vi "PID_auto.vi"() -> ()   [LabVIEW 2025]
uses:
  <vilib>/DAQmx/write.llb/DAQmx Write (Analog 1D DBL NChan 1Samp).vi
  <vilib>/DAQmx/read.llb/DAQmx Read (Analog 1D Wfm NChan NSamp).vi
  <vilib>/Analysis/baseanly.llb/Mean (DBL).vi
  <vilib>/DAQmx/create/channels.llb/DAQmx Create Channel (AO-Voltage-Basic).vi
  <vilib>/DAQmx/configure/timing.llb/DAQmx Timing (Sample Clock).vi
  <vilib>/addons/control/pid/pid.llb/PID (DBL).vi
  <vilib>/addons/control/pid/pid.llb/PID Output Rate Limiter (DBL).vi
  <vilib>/DAQmx/miscellaneous.llb/DAQmx Fill In Error Info.vi
  <resource>/objmgr/daqmx.rc
  <vilib>/addons/control/pid/NI_PID_pid.lvlib
  <vilib>/Analysis/NI_AALBase.lvlib
panel:
  out "Waveform Graph":dbl[](graph)
  out "Mass Flow Rate":dbl
  in  "SO-2":bool
  out "Upstream Temperature":dbl
  out "Inlet Temperature":dbl
  out "PID Gains Indicator":T1={"proportional gain (Kc)"=0.16, "integral time (Ti, min)"=0.0, "derivative time (Td, min)"=0.0}
  in  "Send to Target Position":dbl format="%_3g"
  in  "Emergency Valve Control":dbl format="%_3g"
  in  "Control Options":bool[](array[boolean])
  in  "Control Loop STOP":bool
  in  "Ignition":bool
  in  "SO-1":bool
  out "Valve Output Voltage":dbl format="%_3g"
  out "Time (s)":dbl
  out "error out":errorcluster
  in  "Setpoint":dbl
  out "Thrust Sensor":dbl
  out "Valve Position (%)":dbl format="%_3g"
  out "Differential Pressure":dbl
  out "Chamber Pressure":dbl
  out "Inlet Pressure":dbl
  out "Upstream Pressure":dbl
  out "Supply Pressure":dbl
  in  "Filename":path=path "C:/1. Rocket Research Project/CollectedData/Plots/TestingData.lvm"
  in  "Data Collection Enabled":bool=TRUE caption="Enable"
  in  "Data Collection STOP":bool
  in  "rate":dbl=1000.0 format="%0.2f"
  # "DATA COLLECTION"
  # "CONTROL OPERATIONS"
  # "INSTRUMENTATION"
  # "Pressure"
  # "%"
  # "Emergency Control"
  # "V"
  # "V"
  # "Manual Control"
  # "%"
  # "Auto"
  # "Temperature"
  # "Thrust"
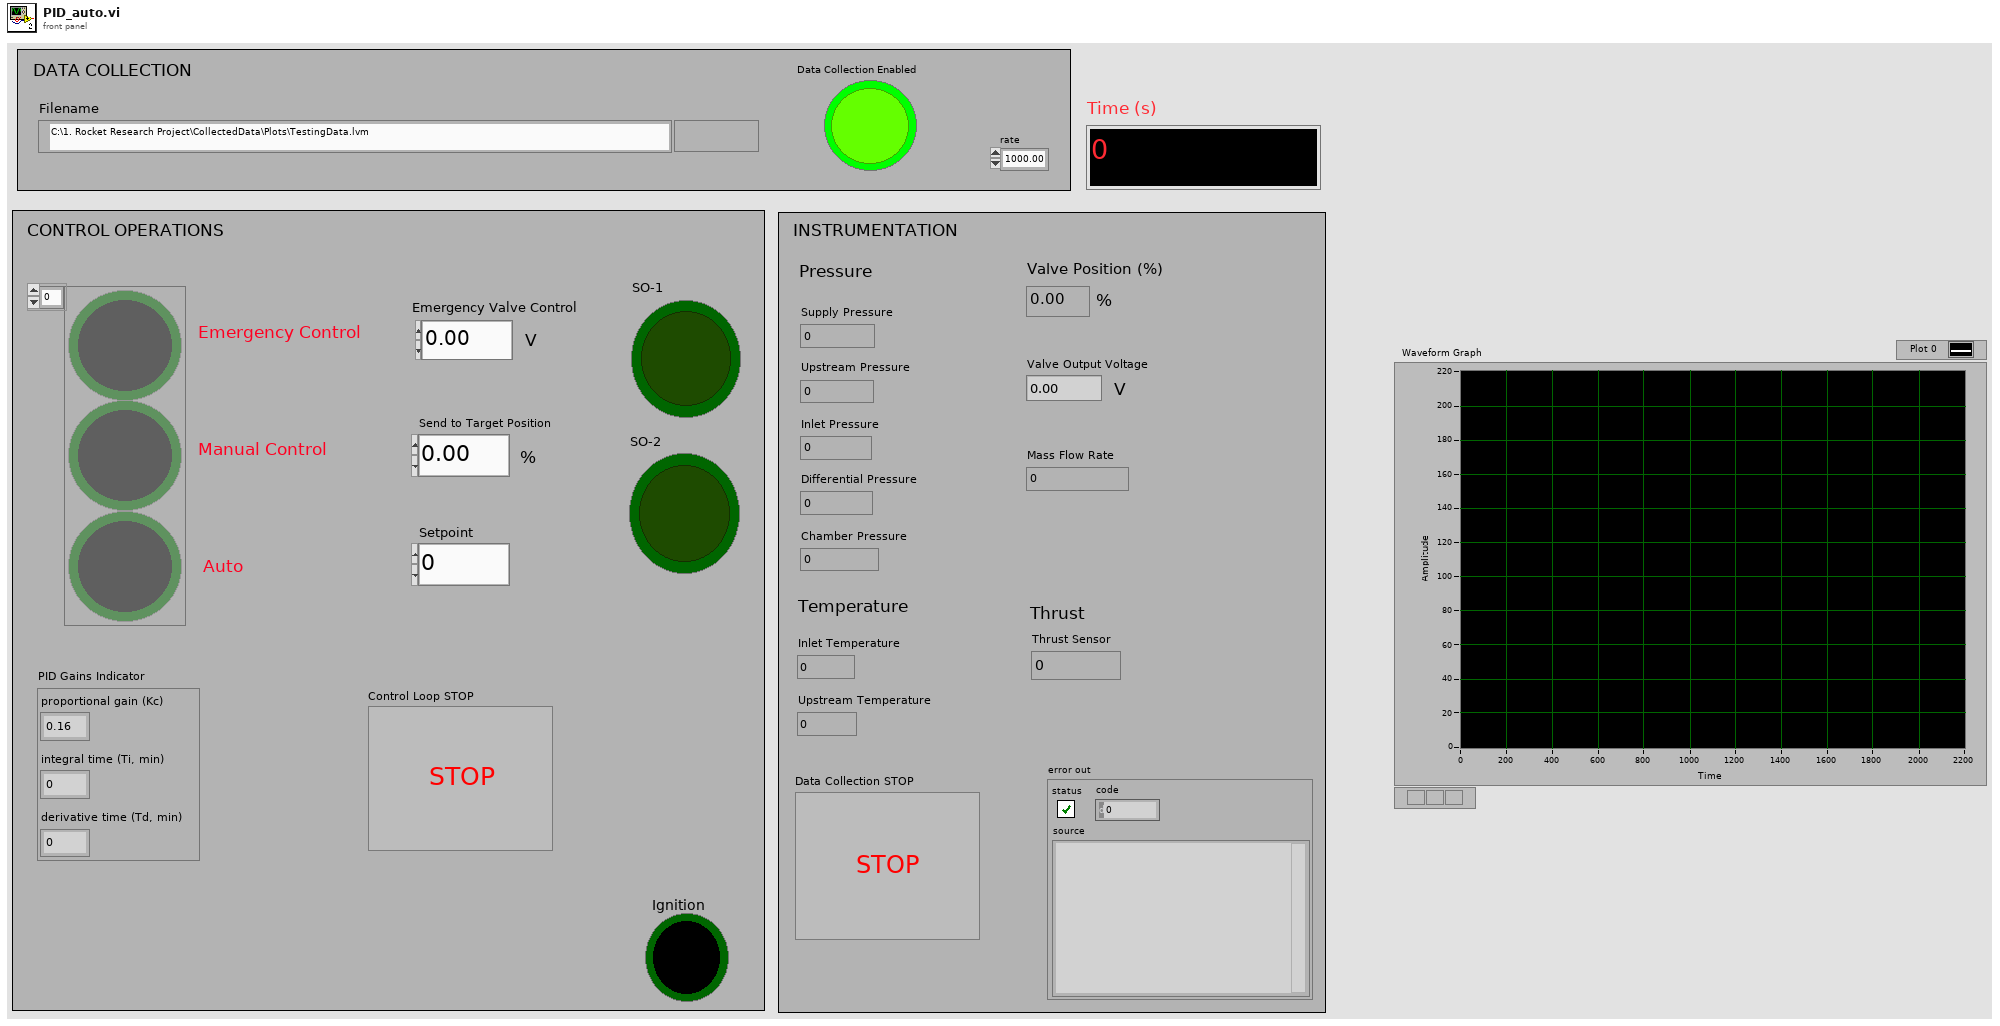
[diagram p1: front panel]
types:
  T1 = cluster{"proportional gain (Kc)":dbl, "integral time (Ti, min)":dbl, "derivative time (Td, min)":dbl}
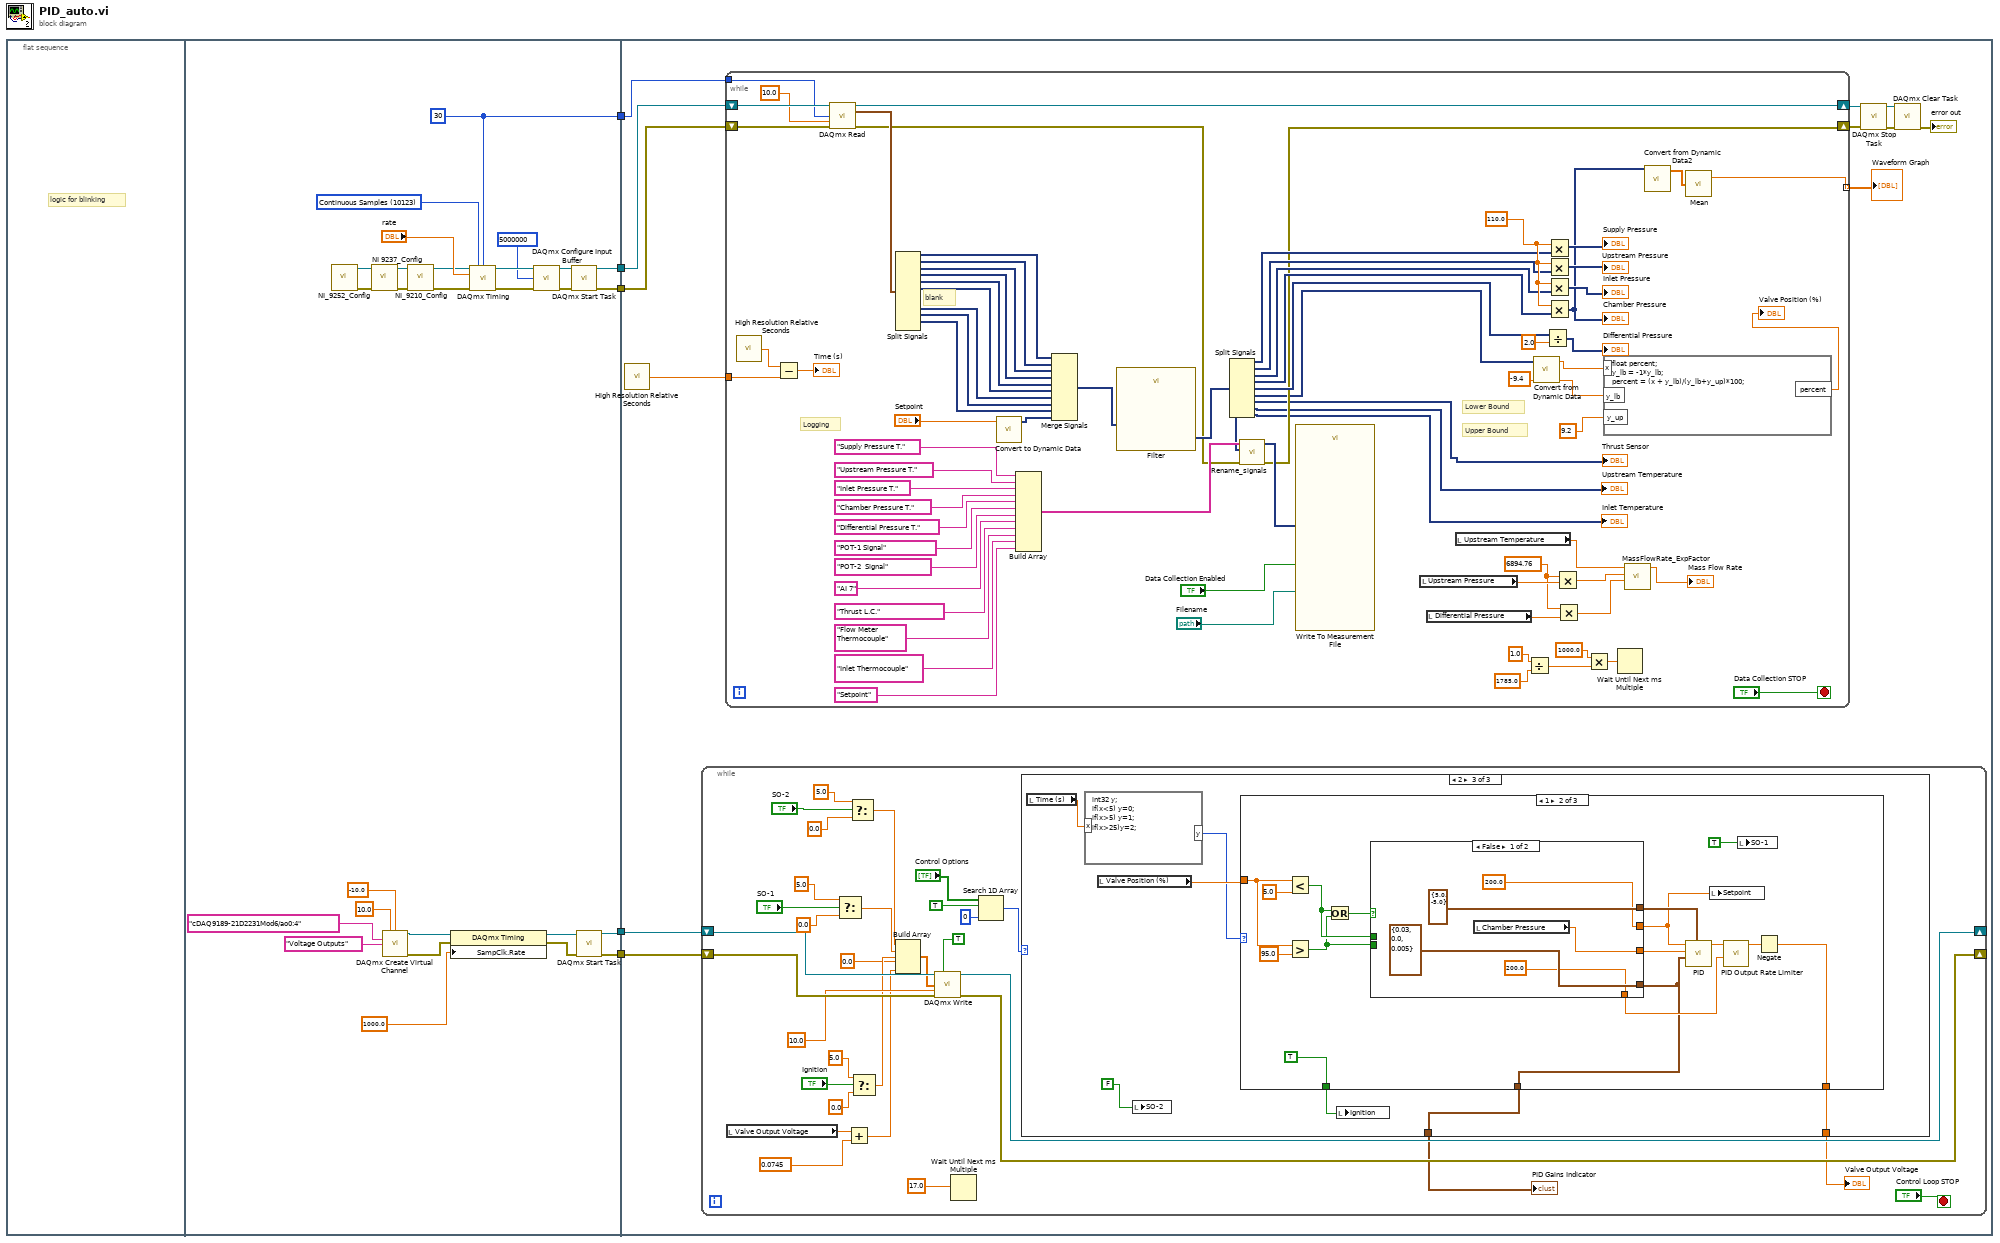
[diagram p0: block diagram]
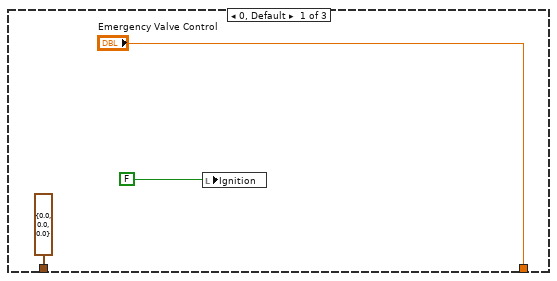
[diagram p2: hidden frame]
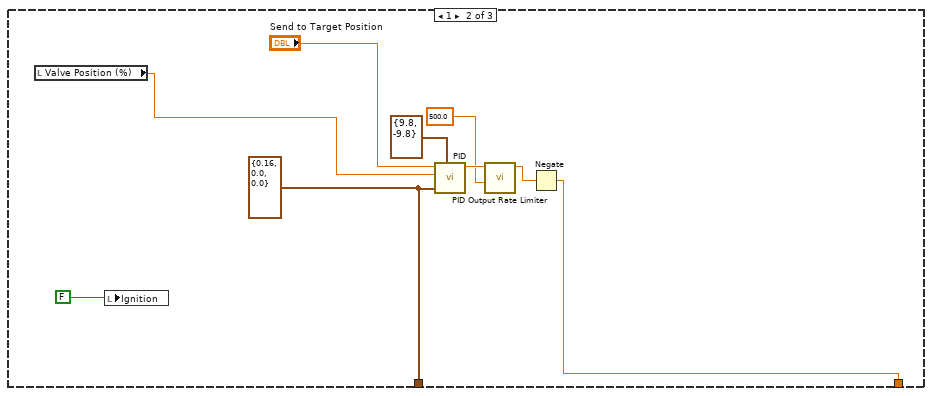
[diagram p3: hidden frame]
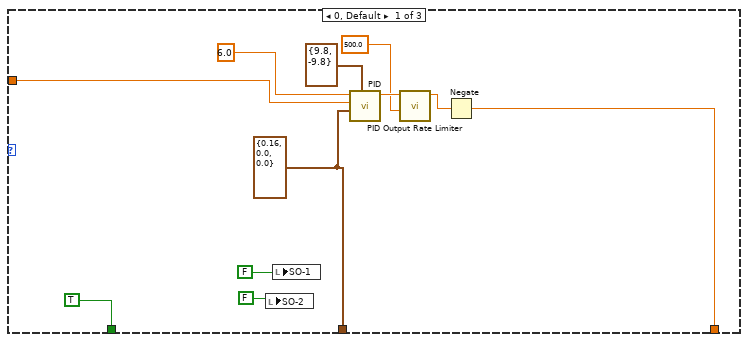
[diagram p4: hidden frame]
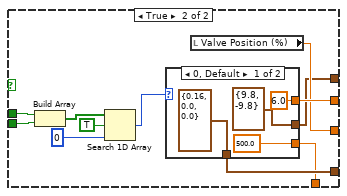
[diagram p5: hidden frame]
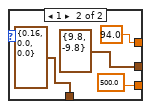
[diagram p6: hidden frame]
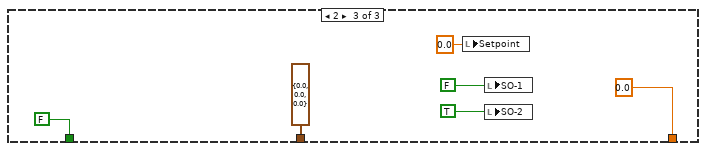
[diagram p7: hidden frame]
diagram:
  n1 = flat-sequence {
    tunnel: [w25] -> w5
    tunnel: [w24] -> w4
    tunnel: [w23] -> w3
    tunnel: [w7] -> w2
    tunnel: [w6] -> w1
    tunnel: w5 -> [w44]
    tunnel: w4 -> [w43]
    tunnel: w3 -> [w42]
    tunnel: w2 -> [w36]
    tunnel: w1 -> [w35]
    frame #0 {
      # "logic for blinking"
    }
    frame #1 {
      w23 = 30 ("samples per channel")
      w32 = 10123 items=["Finite Samples"=10178, "Continuous Samples"=10123, "Hardware Timed Single Point"=12522] ("sample mode")
      n2 = call "NI_9252_Config.vi"() -> ("error out"=w17:errorcluster, "task out"=w18:refnum<k21>)  [unwired: 10 in]
      n3 = call "NI 9237_Config.vi"("error in"=w17, "task in"=w18) -> ("error out"=w20:errorcluster, "task out"=w19:refnum<k21>)  [unwired: 8 in]
      n4 = call-poly <vilib>:"DAQmx Create Virtual Channel.vi"("maximum value"=10.0, "minimum value"=-10.0, "physical channels"="cDAQ9189-21D2231Mod6/ao0:4", "name to assign"="Voltage Outputs") -> ("task out"=w12:refnum<k21>, "error out"=w11:errorcluster)  [unwired: 10 in]
      n5 = call "NI_9210_Config.vi"("error in"=w20, "task in"=w19) -> ("error out"=w21:errorcluster, "task out"=w22:refnum<k21>)  [unwired: 8 in]
      n6 = property class="DAQmx Timing"(reference=w12, error in=w11, "SampClk.Rate"=1000.0) -> (reference out=w10:refnum<k21>, error out=w9:errorcluster)
      n7 = call-poly <vilib>:"DAQmx Timing.vi"("task/channels in"=w22, "sample mode"=w32, "samples per channel"=w23, "rate"="rate", "error in"=w21) -> ("task out"=w30:refnum<k21>, "error out"=w29:errorcluster)  [unwired: 9 in]
      n8 = call <vilib>:"DAQmx Configure Input Buffer.vi"("task/channels in"=w30, "buffer size (in samples per channel)"=u32 5000000, "error in"=w29) -> ("task out"=w27:refnum<k21>, "error out"=w26:errorcluster)  [unwired: 11 in]
      n9 = call <vilib>:"DAQmx Start Task.vi"("task/channels in"=w27, "error in"=w26) -> ("task out"=w25:refnum<k21>, "error out"=w24:errorcluster)  [unwired: 12 in]
      n10 = call <vilib>:"DAQmx Start Task.vi"("task/channels in"=w10, "error in"=w9) -> ("task out"=w7:refnum<k21>, "error out"=w6:errorcluster)  [unwired: 12 in]
    }
    frame #2 {
      n11 = call <vilib>:"High Resolution Relative Seconds.vi"() -> ("relative seconds"=w34:dbl)
      n12 = while {
        shift-right: [w70] -> _
        shift-left: w36 -> [w75]
        shift-right: [w69] -> _
        shift-left: w35 -> [w74]
        stop <- "Control Loop STOP" stop-if-true
        n13 = local read "Valve Output Voltage"() -> (w60:dbl)
        n14 = Select(t=5.0 ("element"), s="SO-1", f=0.0 ("element")) -> (s? t:f=w62:dbl)
        n15 = Add(x=w60, y=0.0745 ("x")) -> (x+y=w58:dbl)
        n16 = Select(t=5.0 ("element"), s="SO-2", f=0.0 ("element")) -> (s? t:f=w48:dbl)
        n17 = Select(t=5.0 ("element"), s="Ignition", f=0.0 ("element")) -> (s? t:f=w61:dbl)
        n18 = Build Array(w48, w62, w61, 0.0 ("element"), w58) -> (w73:dbl[])
        n19 = call-poly <vilib>:"DAQmx Write.vi"("task/channels in"=w75, "auto start"=TRUE, "data"=w73, "timeout"=10.0, "error in"=w74) -> ("task out"=w70:refnum<k21>, "error out"=w69:errorcluster)  [unwired: 8 in, 1 out]
        n20 = Wait Until Next ms Multiple(millisecond multiple=17.0 ("x")) -> ()  [unwired: 1 out]
        n21 = Search 1D Array(1D array="Control Options", element=TRUE ("auto start"), start index (0)=0) -> (index of element=w51:i32)
        n22 = case shown="2" w51 {
          tunnel: ["Emergency Valve Control" w81 w90] -> w50
          tunnel: [T1 {"proportional gain (Kc)"=0.0, "integral time (Ti, min)"=0.0, "derivative time (Td, min)"=0.0} ("PID gains") w79 w89] -> w49
          frame 0, Default {
            n23 = local write "Ignition"(FALSE ("auto start")) -> ()
          }
          frame 1 {
            w79 = T1 {"proportional gain (Kc)"=0.16, "integral time (Ti, min)"=0.0, "derivative time (Td, min)"=0.0} ("PID gains")
            n24 = local read "Valve Position (%)"() -> (w82:dbl)
            n25 = local write "Ignition"(FALSE ("auto start")) -> ()
            n26 = call-poly <vilib>:"PID.vi"("output range"=cluster{"output high":dbl, "output low":dbl} {"output high"=9.8, "output low"=-9.8}, "PID gains"=w79, "process variable"=w82, "setpoint"="Send to Target Position") -> ("output"=w86:dbl)  [unwired: 6 in, 1 out]
            n27 = call-poly <vilib>:"PID Output Rate Limiter.vi"("output rate (EGU/min)"=500.0, "input (controller output)"=w86) -> ("output"=w85:dbl)  [unwired: 6 in, 1 out]
            n28 = Negate(x=w85) -> (-x=w81:dbl)
          }
          frame 2 {
            n29 = local read "Time (s)"() -> (w94:dbl)
            n30 = formula code="int32 y;\nif(x<5) y=0;\nif(x>5) y=1;\nif(x>25)y=2;"("x"=w94) -> ("y"=w92:i32)
            n31 = local read "Valve Position (%)"() -> (w93:dbl)
            n32 = local write "SO-2"(FALSE ("Solenoid")) -> ()
            n33 = case shown="1" w92 {
              tunnel: w93 -> [w98 w121 _]
              tunnel: [w99 w109 0.0 ("element")] -> w90
              tunnel: [TRUE ("Solenoid") TRUE ("Solenoid") FALSE ("Solenoid")] -> w91
              tunnel: [w96 w106 T1 {"proportional gain (Kc)"=0.0, "integral time (Ti, min)"=0.0, "derivative time (Td, min)"=0.0} ("PID gains")] -> w89
              frame 0, Default {
                w96 = T1 {"proportional gain (Kc)"=0.16, "integral time (Ti, min)"=0.0, "derivative time (Td, min)"=0.0} ("PID gains")
                n34 = local write "SO-2"(FALSE ("Solenoid")) -> ()
                n35 = local write "SO-1"(FALSE ("Solenoid")) -> ()
                n36 = call-poly <vilib>:"PID.vi"("output range"=cluster{"output high":dbl, "output low":dbl} {"output high"=9.8, "output low"=-9.8}, "PID gains"=w96, "process variable"=w98, "setpoint"=6.0) -> ("output"=w104:dbl)  [unwired: 6 in, 1 out]
                n37 = call-poly <vilib>:"PID Output Rate Limiter.vi"("output rate (EGU/min)"=500.0, "input (controller output)"=w104) -> ("output"=w103:dbl)  [unwired: 6 in, 1 out]
                n38 = Negate(x=w103) -> (-x=w99:dbl)
              }
              frame 1 {
                n39 = Less?(x=w121, y=5.0 ("element")) -> (x < y?=w111:bool)
                n40 = Greater?(x=w121, y=95.0 ("element")) -> (0:w110:bool)
                n41 = Or(x=w111, y=w110) -> (x .or. y?=w112:bool)
                n42 = case shown="False" w112 {
                  tunnel: w111 -> [_ w137]
                  tunnel: w110 -> [_ w133]
                  tunnel: [T1 {"proportional gain (Kc)"=0.03, "integral time (Ti, min)"=0.0, "derivative time (Td, min)"=0.005} ("PID gains") w131] -> w106
                  tunnel: [200.0 ("element") w130] -> w120
                  tunnel: [200.0 ("element") w129] -> w117
                  tunnel: [w124 w128] -> w119
                  tunnel: [cluster{"output high":dbl, "output low":dbl} {"output high"=5.0, "output low"=-5.0} ("output range") w127] -> w118
                  frame False {
                    n43 = local read "Chamber Pressure"() -> (w124:dbl)
                  }
                  frame True {
                    n44 = Build Array(w137, w133) -> (w136:bool[])
                    n45 = Search 1D Array(1D array=w136, element=TRUE, start index (0)=0) -> (index of element=w132:i32)
                    n46 = case shown="0, Default" w132 {
                      tunnel: [T1 {"proportional gain (Kc)"=0.16, "integral time (Ti, min)"=0.0, "derivative time (Td, min)"=0.0} ("PID gains") T1 {"proportional gain (Kc)"=0.16, "integral time (Ti, min)"=0.0, "derivative time (Td, min)"=0.0} ("PID gains")] -> w131
                      tunnel: [500.0 ("output rate (EGU/min)") 500.0 ("output rate (EGU/min)")] -> w130
                      tunnel: [6.0 ("setpoint") 94.0 ("setpoint")] -> w129
                      tunnel: [cluster{"output high":dbl, "output low":dbl} {"output high"=9.8, "output low"=-9.8} ("output range") cluster{"output high":dbl, "output low":dbl} {"output high"=9.8, "output low"=-9.8} ("output range")] -> w127
                      frame 0, Default {
                      }
                      frame 1 {
                      }
                    }
                    n47 = local read "Valve Position (%)"() -> (w128:dbl)
                  }
                }
                n48 = call-poly <vilib>:"PID.vi"("output range"=w118, "PID gains"=w106, "process variable"=w119, "setpoint"=w117) -> ("output"=w116:dbl)  [unwired: 6 in, 1 out]
                n49 = local write "Setpoint"(w117) -> ()
                n50 = call-poly <vilib>:"PID Output Rate Limiter.vi"("output rate (EGU/min)"=w120, "input (controller output)"=w116) -> ("output"=w115:dbl)  [unwired: 6 in, 1 out]
                n51 = local write "SO-1"(TRUE ("Solenoid")) -> ()
                n52 = Negate(x=w115) -> (-x=w109:dbl)
              }
              frame 2 {
                n53 = local write "Setpoint"(0.0 ("Setpoint")) -> ()
                n54 = local write "SO-1"(FALSE ("Solenoid")) -> ()
                n55 = local write "SO-2"(TRUE ("Solenoid")) -> ()
              }
            }
            n56 = local write "Ignition"(w91) -> ()
          }
        }
        "Valve Output Voltage" <- w50
        "PID Gains Indicator" <- w49
      }
      n57 = while {
        shift-right: [w186] -> w40
        shift-left: w43 -> [w224]
        shift-right: [w221] -> w41
        shift-left: w44 -> [w225]
        tunnel: w42 -> [w223]
        tunnel: w34 -> [w176]
        tunnel: [w152] -> w33 mode=indexing
        stop <- "Data Collection STOP" stop-if-true
        w161 = 6894.76 ("x")
        w219 = 110.0 ("x")
        # "Logging"
        # "blank"
        # "Upper Bound"
        # "Lower Bound"
        n58 = call <vilib>:"High Resolution Relative Seconds.vi"() -> ("relative seconds"=w177:dbl)
        n59 = Subtract(x=w177, y=w176) -> (x-y=→"Time (s)":dbl)
        n60 = call-poly <vilib>:"DAQmx Read.vi"("task/channels in"=w225, "number of samples per channel"=w223, "timeout"=10.0, "error in"=w224) -> ("task out"=w221:refnum<k21>, "data"=w220:waveform(dbl)[], "error out"=w187:errorcluster)  [unwired: 9 in]
        n61 = Split Signals(w220) -> (w168:dynamicdata, w212:dynamicdata, w211:dynamicdata, w209:dynamicdata, w210:dynamicdata, w213:dynamicdata, w165:dynamicdata, w164:dynamicdata, w163:dynamicdata)  [unwired: 12 in, 3 out]
        n62 = call "Convert to Dynamic Data"("Double"="Setpoint") -> ("Dynamic Data Type"=w183:dynamicdata)  [unwired: 3 in]
        n63 = Build Array("Supply Pressure T.", "Upstream Pressure T.", "Inlet Pressure T.", "Chamber Pressure T.", "Differential Pressure T.", "POT-1 Signal", "POT-2  Signal", "AI 7" ("element"), "Thrust L.C.", "Flow Meter Thermocouple", "Inlet Thermocouple", "Setpoint" ("element")) -> (w196:string[])
        n64 = Merge Signals(w168, w212, w211, w209, w210, w213, w165, w164, w163, w183) -> (w194:dynamicdata)
        n65 = call "Filter"("Signal"=w194) -> ("Filtered Signal"=w193:dynamicdata)  [unwired: 9 in, 1 out]
        n66 = Split Signals(w193) -> (w192:dynamicdata, w191:dynamicdata, w190:dynamicdata, w189:dynamicdata, w188:dynamicdata, w173:dynamicdata, →"Thrust Sensor":dynamicdata, →"Upstream Temperature":dynamicdata, →"Inlet Temperature":dynamicdata)  [unwired: 9 in]
        n67 = call "Rename_signals.vi"("error in"=w187, "Dynamic Data In"=w193, "New Signal Names"=w196) -> ("error out"=w186:errorcluster, "Dynamic Data Out"=w195:dynamicdata)  [unwired: 7 in]
        n68 = call "Write To Measurement File"("Signals"=w195, "Enable"="Data Collection Enabled", "Filename"="Filename") -> ()  [unwired: 14 in, 3 out]
        n69 = local read "Upstream Pressure"() -> (w162:dbl)
        n70 = local read "Differential Pressure"() -> (w160:dbl)
        n71 = local read "Upstream Temperature"() -> (w156:dbl)
        n72 = Divide(x=1.0, y=1785.0 ("x")) -> (x/y=w181:dbl)
        n73 = call "Convert from Dynamic Data"("Dynamic Data Type"=w173) -> ("Scalar"=w172:dbl)  [unwired: 3 in]
        n74 = Divide(x=w188, y=2.0) -> (x/y=→"Differential Pressure":dynamicdata)
        n75 = Multiply(x=w219, y=w192) -> (x*y=→"Supply Pressure":dynamicdata)
        n76 = Multiply(x=w219, y=w191) -> (x*y=→"Upstream Pressure":dynamicdata)
        n77 = Multiply(x=w219, y=w190) -> (x*y=→"Inlet Pressure":dynamicdata)
        n78 = Multiply(x=w219, y=w189) -> (x*y=w154:dynamicdata)
        "Chamber Pressure" <- w154
        n79 = Multiply(x=w161, y=w162) -> (x*y=w158:dbl)
        n80 = Multiply(x=w161, y=w160) -> (x*y=w157:dbl)
        n81 = Multiply(x=1000.0, y=w181) -> (x*y=w180:dbl)
        n82 = formula code="float percent;\ny_lb = -1*y_lb;\npercent = (x + y_lb)/(y_lb+y_up)*100;"("x"=w172, "y_lb"=-9.4 ("y"), "y_up"=9.2 ("y")) -> ("percent"=→"Valve Position (%)":dbl)
        n83 = Wait Until Next ms Multiple(millisecond multiple=w180) -> ()  [unwired: 1 out]
        n84 = call "MassFlowRate_ExpFactor.vi"("Differential Pressure"=w157, "Upstream Pressure"=w158, "Upstream \nTemperature"=w156) -> ("Mass Flow Rate"=→"Mass Flow Rate":dbl)  [unwired: 8 in]
        n85 = call "Convert from Dynamic Data2"("Dynamic Data Type"=w154) -> ("Array"=w153:dbl[])  [unwired: 3 in]
        n86 = call-poly <vilib>:"Mean.vi"("X"=w153) -> ("mean"=w152:dbl)  [unwired: 1 out]
      }
      "Waveform Graph" <- w33
      n87 = call <vilib>:"DAQmx Stop Task.vi"("task/channels in"=w41, "error in"=w40) -> ("task out"=w39:refnum<k21>, "error out"=w38:errorcluster)  [unwired: 12 in]
      n88 = call <vilib>:"DAQmx Clear Task.vi"("task in"=w39, "error in"=w38) -> ("error out"=→"error out":errorcluster)  [unwired: 13 in]
    }
  }
